vi "Handle Message.vi"(8 "error in (no error)":errorcluster, 9 "Message Completion Handler":refnum<class "Message Completion Handler.lvclass">, 10 "Message":string, 11 "Plugin In":refnum<class "Sift TDMS Uploader.lvclass">) -> (0 "error out":errorcluster, 1 "Synchronously Complete Message?":bool=TRUE, 2 "Message Response":string, 3 "Plugin out":refnum<class "Sift TDMS Uploader.lvclass">)   [LabVIEW 2024, in "Sift TDMS Uploader.lvlib" / "Sift TDMS Uploader.lvclass"]
uses:
  Sift TDMS Uploader.lvclass
  <vilib>/FlexLogger/SDK/PluginSDK.lvlibp/PEFClasses/SDK/Message Completion Handler/Message Completion Handler.lvclass
  Sift TDMS Uploader.lvclass/Sift TDMS Uploader.ctl
  SubVIs/Log Event Types.ctl
  Globals.vi
  <vilib>/FlexLogger/SDK/PluginSDK.lvlibp/PEFClasses/SDK/Processing Element/Read System Interface.vi
  <vilib>/FlexLogger/SDK/PluginSDK.lvlibp/PEFClasses/SDK/Processing Element/Read Alias.vi
  <vilib>/FlexLogger/SDK/PluginSDK.lvlibp/PEFClasses/SDK/System Interface/System Interface.lvclass
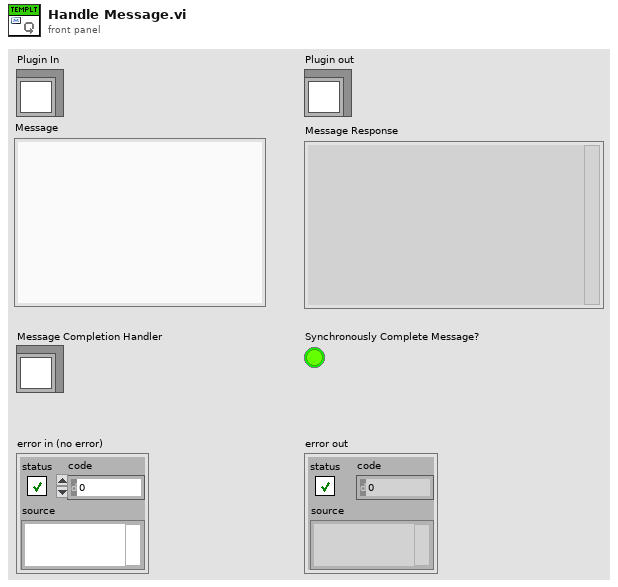
[diagram p1: front panel]
types:
  T1 = typedef "Sift TDMS Uploader.lvlib/Sift TDMS Uploader.lvclass/Log Event Types.ctl" = enum16{"INFO", "WARN", "ERROR"}
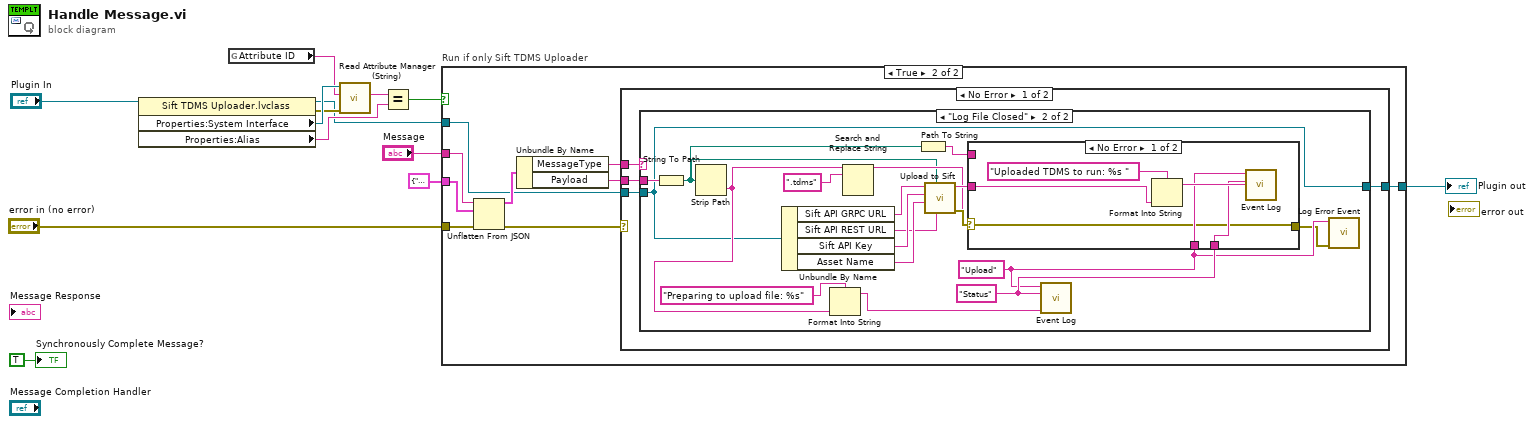
[diagram p0: block diagram]
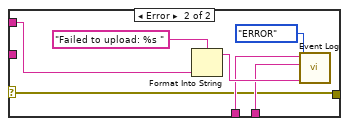
[diagram p4: hidden frame]
diagram:
  n1 = property class="Sift TDMS Uploader.lvclass"(reference="Plugin In") -> (reference out=w1:refnum<class "Sift TDMS Uploader.lvclass">, error out=w11:errorcluster, "Properties:System Interface"=w12:refnum<class "System Interface.lvclass">, "Properties:Alias"=w3:string)  [unwired: 1 in]
  n2 = global read "Globals.vi" "Attribute ID"() -> (w10:string)
  n3 = call-dynamic "Read Attribute Manager (String).vi"("error in (no error)"=w11, "Attribute ID"=w10, "System Interface in"=w12) -> ("Attrib Val"=w4:string)  [unwired: 5 in, 3 out]
  n4 = Equal?(x=w4, y=w3) -> (x = y?=w9:bool)
  n5 = case "Run if only Sift TDMS Uploader" shown="True" w9 {
    tunnel: w1 -> [w14 w19]
    tunnel: "Message" -> [_ w18]
    tunnel: cluster{"Payload":string, "MessageType":string} {"Payload"="", "MessageType"=""} -> [_ w17]
    tunnel: "error in (no error)" -> [_ w16]
    tunnel: [w14 w15] -> w5
    frame False {
    }
    frame True {
      n6 = Unflatten From JSON(JSON string=w18, type and defaults=w17, error in (no error)=w16) -> (value=w20:cluster{"Payload":string, "MessageType":string}, error out=w21:errorcluster)  [unwired: 4 in]
      n7 = Unbundle By Name(w20) -> ("MessageType"=w22:string, "Payload"=w23:string)
      n8 = case shown="No Error" w21 {
        tunnel: w22 -> [w27 _]
        tunnel: w23 -> [w25 _]
        tunnel: w19 -> [w26 w60]
        tunnel: [w24 w60] -> w15
        frame No Error {
          n9 = case shown="\"Log File Closed\"" w27 {
            tunnel: w25 -> [_ w46]
            tunnel: w26 -> [w28 w34]
            tunnel: [w28 w34] -> w24
            frame Default {
            }
            frame "Log File Closed" {
              w33 = "Status"
              w30 = "Upload"
              n10 = String To Path(string=w46) -> (path=w32:path)
              n11 = Strip Path(path=w32) -> (name=w36:string)  [unwired: 1 out]
              n12 = Unbundle By Name(w34) -> ("Sift API GRPC URL"=w45:string, "Sift API REST URL"=w42:string, "Sift API Key"=w44:string, "Asset Name"=w43:string)
              n13 = Format Into String(format string="Preparing to upload file: %s", w36) -> (resulting string=w35:string)  [unwired: 2 in, 1 out]
              n14 = Search and Replace String(input string=w36, search string=".tdms") -> (result string=w39:string)  [unwired: 6 in, 3 out]
              n15 = Path To String(path=w32) -> (string=w31:string)
              n16 = call "Upload to Sift.vi"("API REST URL"=w42, "Absolute Filepath"=w32, "Run Name"=w39, "Asset Name"=w43, "API Key"=w44, "API GRPC URL"=w45) -> ("Error"=w40:errorcluster, "Run URL"=w41:string)  [unwired: 4 in]
              n17 = case shown="No Error" w40 {
                selector: w40 -> [w47 w54]
                tunnel: w41 -> [w51 _]
                tunnel: w30 -> [w49 w55]
                tunnel: w33 -> [w48 w56]
                tunnel: w31 -> [_ w53]
                tunnel: [w47 w54] -> w29
                frame No Error {
                  n18 = Format Into String(format string="Uploaded TDMS to run: %s ", w51) -> (resulting string=w50:string)  [unwired: 2 in, 1 out]
                  n19 = call "Event Log.vi"("Message"=w50, "Event Type"=w48, "Location"=w49) -> ()  [unwired: 9 in]
                }
                frame Error {
                  n20 = Format Into String(format string="Failed to upload: %s ", w53) -> (resulting string=w58:string)  [unwired: 2 in, 1 out]
                  n21 = call "Event Log.vi"("Message"=w58, "Log Event Type"=Log_Event_Types."ERROR" ("Log Event Types"), "Event Type"=w56, "Location"=w55) -> ()  [unwired: 8 in]
                }
              }
              n22 = call "Event Log.vi"("Message"=w35, "Event Type"=w33, "Location"=w30) -> ()  [unwired: 9 in]
              n23 = call "Log Error Event.vi"("error in (no error)"=w29, "Location"=w30) -> ()  [unwired: 10 in]
            }
          }
        }
        frame Error {
        }
      }
    }
  }
  "Plugin out" <- w5
  "Synchronously Complete Message?" <- TRUE ("Synchronously Complete Message?")
